vi "TCP Client_31.vi"(0 "remote port or service name":u16, 1 "Cmd":i8, 2 "Data":string, 3 "error in (no error)":errorcluster, 4 "Address":string, 5 "timeout ms":i32) -> (6 "R_message 1":string, 7 "error out":errorcluster)   [LabVIEW 2022 SP3]
panel:
  out "R_message 2":string
  out "R_Data string length":cluster{i32}
  out "W_Data string length: \nbytes written 2":i32
  out "W_Data string_flat":string
  # "send= 11 / 8 / 9"
  # "9 = signals\n8 = data2Matrix"
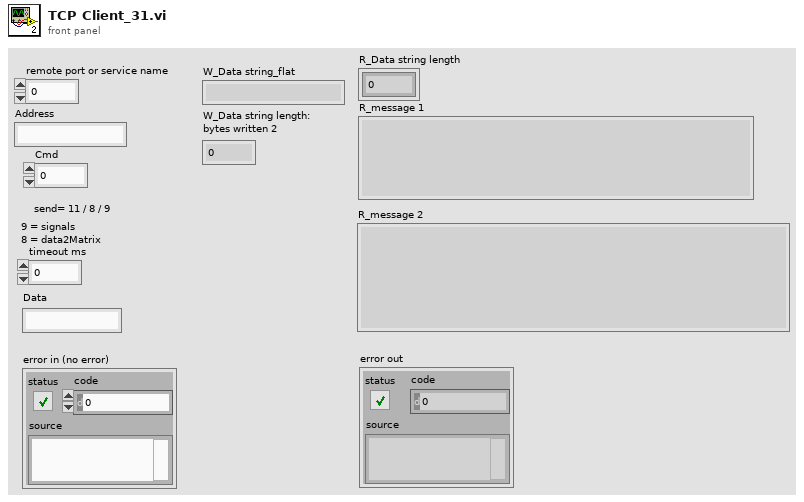
[diagram p1: front panel]
types:
  T1 = enum16{"big-endian, network order", "native, host order", "little-endian"}
  T2 = enum16{"Standard", "Buffered", "CRLF", "Immediate"}
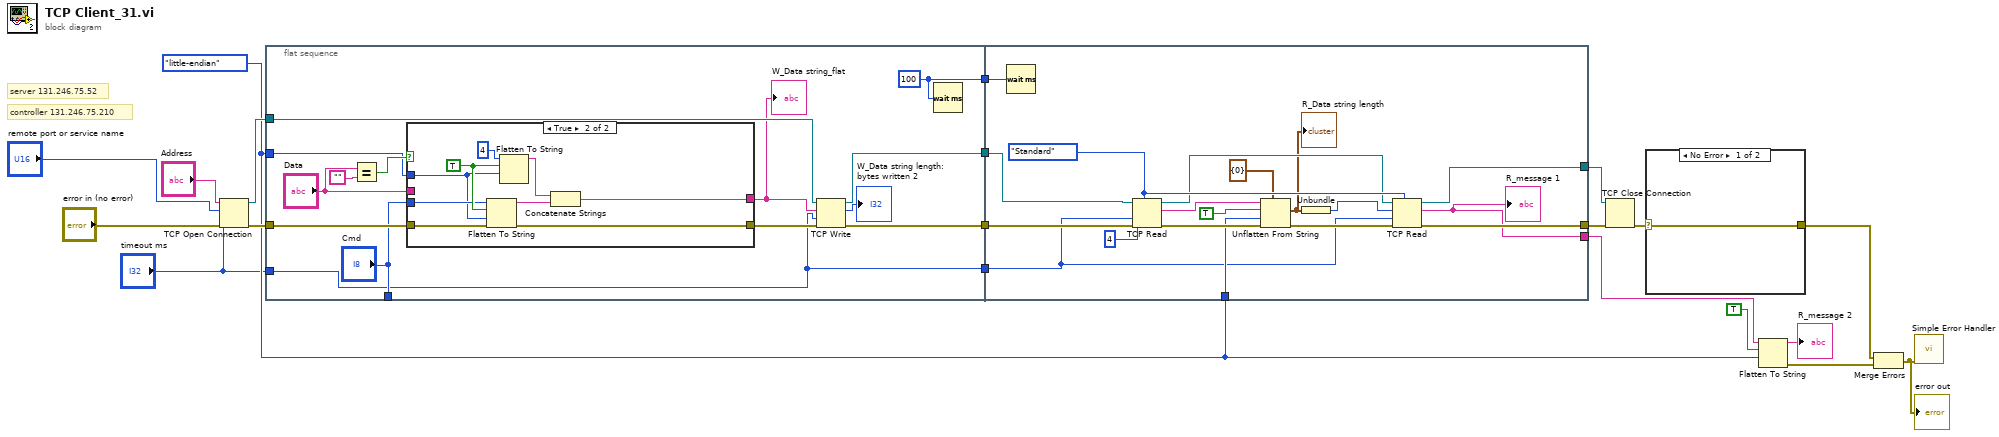
[diagram p0: block diagram]
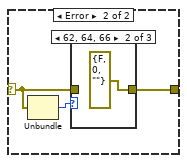
[diagram p2: hidden frame]
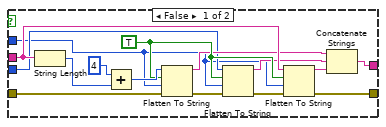
[diagram p5: hidden frame]
diagram:
  w4 = T1."little-endian" ("byte order (0:big-endian, network order)")
  # "controller 131.246.75.210"
  # "server 131.246.75.52"
  n1 = TCP Open Connection(address="Address", remote port or service name="remote port or service name", timeout ms (60000)="timeout ms", error in (no error)="error in (no error)") -> (connection ID=w18:refnum<k5>, error out=w17:errorcluster)  [unwired: 1 in]
  n2 = flat-sequence {
    tunnel: w18 -> [w33]
    tunnel: w17 -> [w26]
    tunnel: [w32] -> w16
    tunnel: [w31] -> w15
    tunnel: [w30] -> w9
    tunnel: w4 -> [w23]
    tunnel: ["Cmd"] -> _
    tunnel: "timeout ms" -> [w21]
    tunnel: [w21] -> w1
    tunnel: w16 -> [w74]
    tunnel: w15 -> [w73]
    tunnel: [w60] -> w8
    tunnel: [w72] -> w11
    tunnel: [w71] -> w10
    tunnel: w9 -> [w63]
    tunnel: w4 -> [w62]
    tunnel: w1 -> [w59]
    frame #0 {
      w30 = u32 100 ("milliseconds to wait")
      n3 = Equal?(x="Data", y="") -> (x = y?=w28:bool)
      n4 = case shown="True" w28 {
        tunnel: "Data" -> [w46 _]
        tunnel: w26 -> [w41 w58]
        tunnel: [w38 w57] -> w25
        tunnel: [w37 w54] -> w24
        tunnel: "Cmd" -> [w36 w51]
        tunnel: w23 -> [w35 w50]
        frame False {
          w45 = TRUE ("prepend array or string size? (T)")
          n5 = String Length(string=w46) -> (length=w48:i32)
          n6 = Add(x=4, y=w48) -> (x+y=w47:i32)
          n7 = Flatten To String(anything=w47, prepend array or string size? (T)=w45, byte order (0:big-endian, network order)=w35, error in (no error)=w41) -> (data string=w44:string, error out=w40:errorcluster)  [unwired: 1 out]
          n8 = Flatten To String(anything=w36, prepend array or string size? (T)=w45, byte order (0:big-endian, network order)=w35, error in (no error)=w40) -> (data string=w43:string, error out=w39:errorcluster)  [unwired: 1 out]
          n9 = Flatten To String(anything=w46, prepend array or string size? (T)=w45, byte order (0:big-endian, network order)=w35, error in (no error)=w39) -> (data string=w42:string, error out=w38:errorcluster)  [unwired: 1 out]
          n10 = Concatenate Strings(w44, w43, w42) -> (w37:string)
        }
        frame True {
          w52 = TRUE ("prepend array or string size? (T)")
          n11 = Flatten To String(anything=w51, prepend array or string size? (T)=w52, byte order (0:big-endian, network order)=w50, error in (no error)=w58) -> (data string=w55:string, error out=w57:errorcluster)  [unwired: 1 out]
          n12 = Flatten To String(anything=4, prepend array or string size? (T)=w52, byte order (0:big-endian, network order)=w50) -> (data string=w56:string)  [unwired: 1 in, 2 out]
          n13 = Concatenate Strings(w56, w55) -> (w54:string)
        }
      }
      "W_Data string_flat" <- w24
      n14 = TCP Write(connection ID=w33, data in=w24, error in (no error)=w25, 9:w21) -> (connection ID out=w31:refnum<k5>, bytes written=→"W_Data string length: \nbytes written 2":i32, error out=w32:errorcluster)
      n15 = Wait (ms)(milliseconds to wait=w30) -> ()  [unwired: 1 out]
    }
    frame #1 {
      w76 = T2."Standard" ("mode (standard)")
      n16 = Wait (ms)(milliseconds to wait=w63) -> ()  [unwired: 1 out]
      n17 = TCP Read(connection ID=w73, bytes to read=4, error in (no error)=w74, 7:w76, 9:w59) -> (connection ID out=w75:refnum<k5>, data out=w70:string, error out=w65:errorcluster)
      n18 = Unflatten From String(type=cluster{i32} {0}, binary string=w70, data includes array or string size? (T)=TRUE, byte order (0:big-endian, network order)=w62, error in (no error)=w65) -> (value=w67:cluster{i32}, error out=w64:errorcluster)  [unwired: 1 out]
      "R_Data string length" <- w67
      n19 = Unbundle(w67) -> (w66:i32)
      n20 = TCP Read(connection ID=w75, bytes to read=w66, error in (no error)=w64, 7:w76, 9:w59) -> (connection ID out=w72:refnum<k5>, data out=w60:string, error out=w71:errorcluster)
      "R_message 1" <- w60
    }
  }
  n21 = TCP Close Connection(connection ID=w11, error in (no error)=w10) -> (error out=w12:errorcluster)  [unwired: 1 in, 1 out]
  n22 = case shown="No Error" w12 {
    selector: w12 -> [w77 w79]
    tunnel: [w77 w78] -> w13
    frame No Error {
    }
    frame Error {
      n23 = Unbundle(w79) -> ("code"=w80:i32)  [unwired: 2 out]
      n24 = case shown="62, 64, 66" w80 {
        tunnel: [w81 errorcluster {"status"=FALSE, "code"=0, "source"=""} ("error IO") w83] -> w78
        tunnel: w79 -> [w81 _ w83]
        frame 0, Default {
        }
        frame 62, 64, 66 {
        }
        frame 56 {
        }
      }
    }
  }
  n25 = Flatten To String(anything=w8, prepend array or string size? (T)=TRUE, byte order (0:big-endian, network order)=w4) -> (data string=→"R_message 2":string, error out=w6:errorcluster)  [unwired: 1 in, 1 out]
  n26 = Merge Errors(w13, w6) -> (w14:errorcluster)
  "error out" <- w14
  n27 = call <vilib>:"Simple Error Handler.vi"("error in (no error)"=w14) -> ()  [unwired: 4 in, 5 out]
